vi "Use FGV2.vi"() -> ()   [LabVIEW 2022 SP3]
panel:
  out "Subscriber 2":dbl
  in  "stop":bool
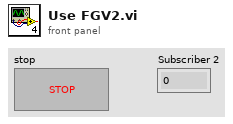
[diagram p1: front panel]
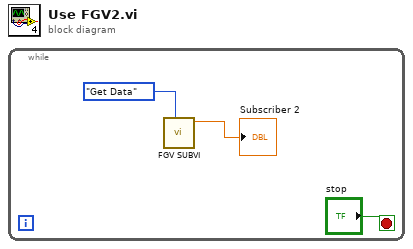
[diagram p0: block diagram]
diagram:
  n1 = while {
    stop <- "stop" stop-if-true
    n2 = call "FGV SUBVI.vi"("Enum"=enum16{"Get Data", "Set Data"}."Get Data") -> ("Data Input out"=→"Subscriber 2":dbl)  [unwired: 10 in]
  }
